vi "CMDExec.vi"() -> ()   [LabVIEW 2012]
uses:
  <vilib>/addons/database/Connection.llb/DB Tools Open Connec (String).vi
  <vilib>/Utility/file.llb/Read From Spreadsheet File (I64).vi
  <vilib>/Utility/file.llb/Read From Spreadsheet File (string).vi
  <vilib>/addons/database/NI_Database_API.lvlib
panel:
  in  "lot_end":string
  in  "lot_start":string
  out "output cluster":T1
  in  "input cluster":T1
  out "before substring 9":string
  out "concatenated string":string
  out "before substring":string
  out "standard output 3":string
  out "after substring":string
  out "text":string
  out "error out":errorcluster
  in  "error in (no error)":errorcluster
  out "standard error 2":string
  out "standard output 2":string
  out "standard error":string
  out "standard output":string
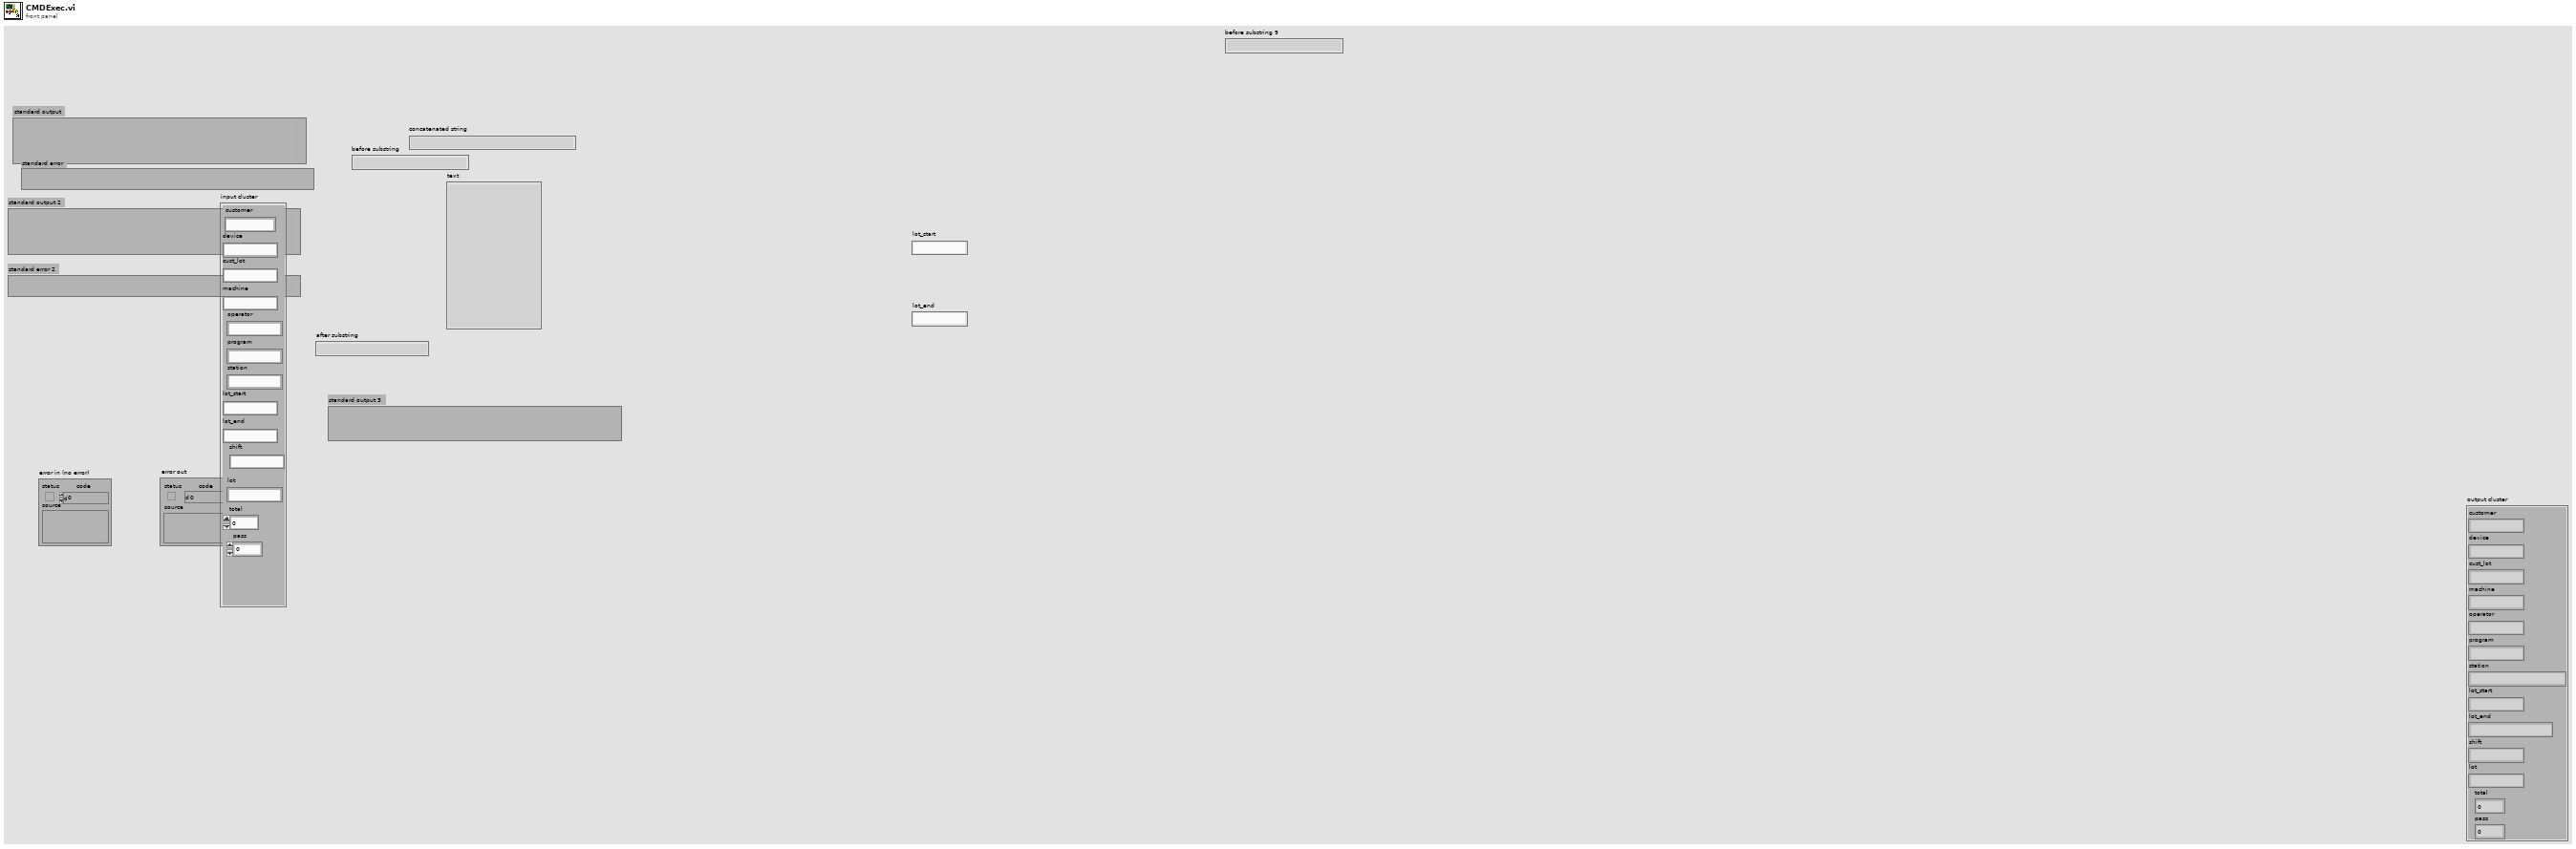
[diagram p1: front panel]
types:
  T1 = cluster{"customer":string, "device":string, "cust_lot":string, "machine":string, "operator":string, "program":string, "station":string, "lot_start":string, "lot_end":string, "shift":string, "lot":string, "total":dbl, "pass":dbl}
  T2 = enum16{"open", "replace", "create", "open or create", "replace or create", "replace or create with confirmation"}
  T3 = typedef "NI_Database_API.lvlib/Conn ObjectReference.ctl" = refnum<k1>
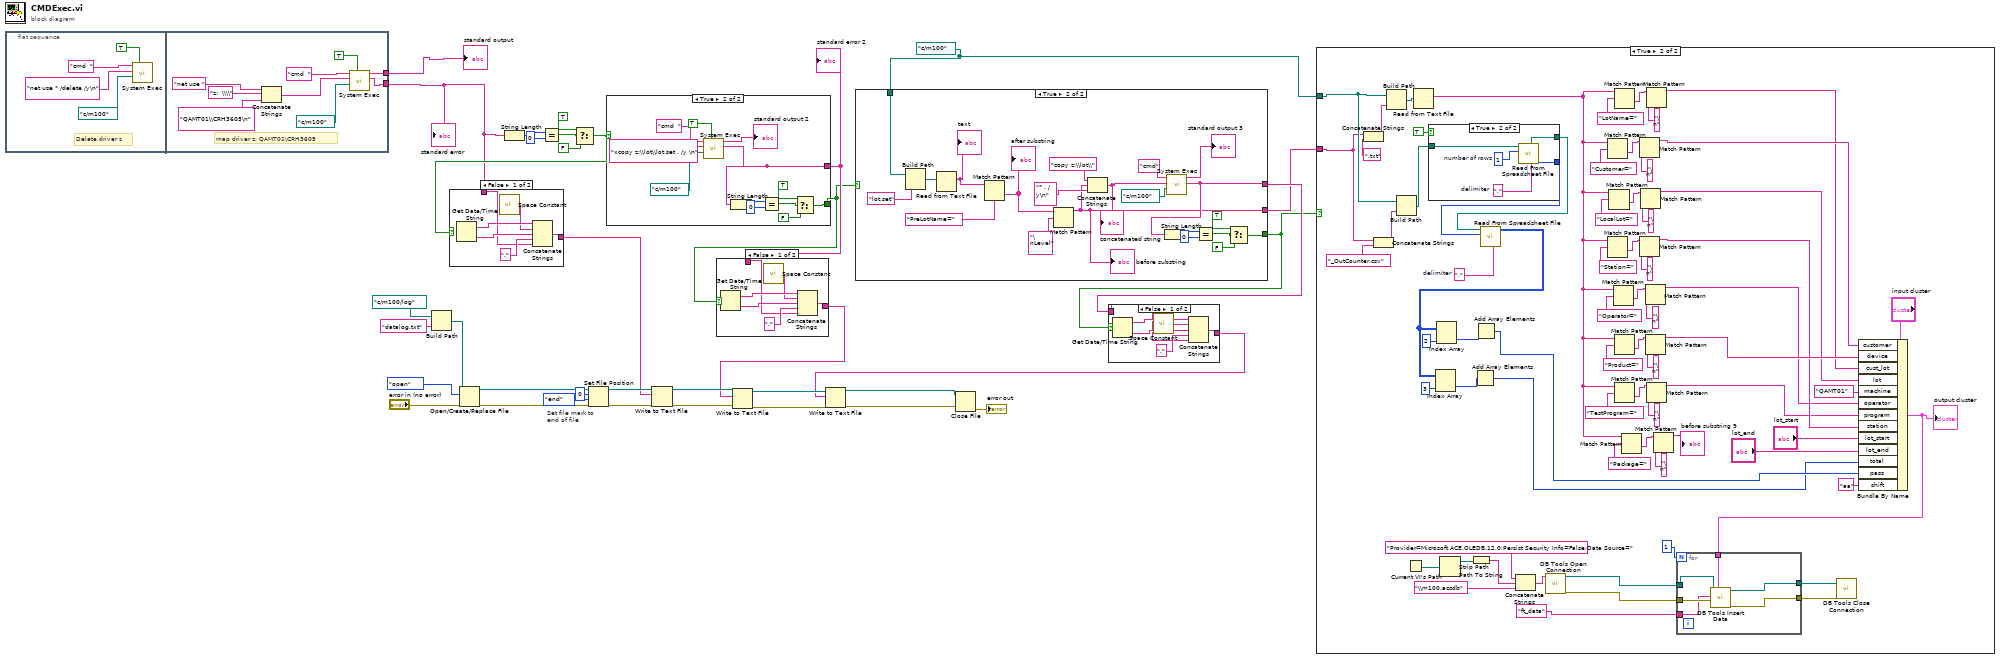
[diagram p0: block diagram]
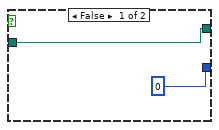
[diagram p3: hidden frame]
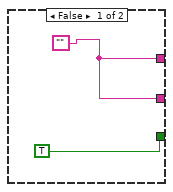
[diagram p5: hidden frame]
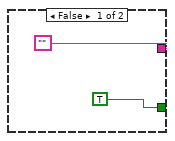
[diagram p8: hidden frame]
diagram:
  w2 = path "c:/m100" ("base path")
  # "Set file mark to\nend of file"
  n1 = flat-sequence {
    tunnel: [w41] -> w12
    tunnel: [w40] -> w11
    frame #0 {
      # "Delete driver z"
      n2 = call <vilib>:"System Exec.vi"("wait until completion? (T)"=TRUE, "working directory"=path "c:/m100", "standard input"="net use * /delete /y\n" ("string"), "command line"="cmd  ") -> ()  [unwired: 2 in, 6 out]
    }
    frame #1 {
      # "map driver z: QAMT01\\CRH3605"
      n3 = Concatenate Strings("net use " ("string"), "z:  \\\\" ("string"), "QAMT01\\CRH3605\n" ("string")) -> (w47:string)
      n4 = call <vilib>:"System Exec.vi"("wait until completion? (T)"=TRUE, "working directory"=path "c:/m100", "standard input"=w47, "command line"="cmd  ") -> ("standard error"=w40:string, "standard output"=w41:string)  [unwired: 2 in, 4 out]
    }
  }
  n5 = Build Path(base path=path "c:/m100/log" ("path"), name or relative path="datalog.txt") -> (appended path=w19:path)
  n6 = Open/Create/Replace File(file path (use dialog)=w19, error in="error in (no error)", operation (0:open)=T2."open") -> (refnum out=w24:refnum<file>, error out=w23:errorcluster)  [unwired: 3 in, 1 out]
  n7 = String Length(string=w11) -> (length=w35:i32)
  n8 = Equal?(x=w35, y=0) -> (x = y?=w33:bool)
  n9 = Select(t=TRUE, s=w33, f=FALSE) -> (s? t:f=w16:bool)
  n10 = case shown="False" w16 {
    tunnel: [w50 w55] -> w14
    tunnel: w11 -> [w49 w55]
    frame False {
      n11 = Get Date/Time String() -> (date string=w52:string, time string=w53:string)  [unwired: 3 in]
      n12 = call <vilib>:"Space Constant.vi"() -> ("String"=w51:string)
      n13 = Concatenate Strings(w52, w51, w53, "," ("string"), w49) -> (w50:string)
    }
    frame True {
    }
  }
  n14 = Set File Position(offset (in bytes) (0)=i64 0, refnum=w24, from (0:start)=enum16{"start", "end", "current"}."end", error in=w23) -> (refnum out=w26:refnum<file>, error out=w27:errorcluster)
  n15 = case shown="True" w16 {
    tunnel: [TRUE w59] -> w10
    tunnel: ["" w58] -> w15
    frame False {
    }
    frame True {
      n16 = call <vilib>:"System Exec.vi"("wait until completion? (T)"=TRUE, "working directory"=path "c:/m100", "standard input"="xcopy z:\\lot\\lot.set . /y \n", "command line"="cmd  ") -> ("standard error"=w58:string, "standard output"=→"standard output 2":string)  [unwired: 2 in, 4 out]
      n17 = String Length(string=w58) -> (length=w65:i32)
      n18 = Equal?(x=w65, y=0) -> (x = y?=w67:bool)
      n19 = Select(t=TRUE, s=w67, f=FALSE) -> (s? t:f=w59:bool)
    }
  }
  "standard error 2" <- w15
  n20 = Write to Text File(file (use dialog)=w26, text=w14, error in=w27) -> (refnum out=w18:refnum<file>, error out=w17:errorcluster)  [unwired: 1 in, 1 out]
  n21 = case shown="False" w10 {
    tunnel: [w71 w76] -> w13
    tunnel: w15 -> [w70 w76]
    frame False {
      n22 = Get Date/Time String() -> (date string=w73:string, time string=w74:string)  [unwired: 3 in]
      n23 = call <vilib>:"Space Constant.vi"() -> ("String"=w72:string)
      n24 = Concatenate Strings(w73, w72, w74, "," ("string"), w70) -> (w71:string)
    }
    frame True {
    }
  }
  n25 = Write to Text File(file (use dialog)=w18, text=w13, error in=w17) -> (refnum out=w6:refnum<file>, error out=w9:errorcluster)  [unwired: 1 in, 1 out]
  n26 = case shown="True" w10 {
    tunnel: [TRUE w83] -> w3
    tunnel: [w77 w82] -> w4
    tunnel: w2 -> [_ w80]
    tunnel: [w77 w79] -> w1
    frame False {
      w77 = ""
    }
    frame True {
      n27 = Build Path(base path=w80, name or relative path="lot.set") -> (appended path=w99:path)
      n28 = Read from Text File(file (use dialog)=w99) -> (text=w96:string)  [unwired: 3 in, 3 out]
      "text" <- w96
      n29 = Match Pattern(string=w96, regular expression="PreLotName=") -> (after substring=w90:string)  [unwired: 1 in, 3 out]
      "after substring" <- w90
      n30 = Match Pattern(string=w90, regular expression="\nLevel") -> (before substring=w79:string)  [unwired: 1 in, 3 out]
      "before substring" <- w79
      n31 = Concatenate Strings("copy z:\\lot\\" ("string"), w79, "* . /y\n" ("string")) -> (w89:string)
      "concatenated string" <- w89
      n32 = call <vilib>:"System Exec.vi"("working directory"=path "c:/m100", "standard input"=w89, "command line"="cmd") -> ("standard error"=w82:string, "standard output"=→"standard output 3":string)  [unwired: 3 in, 4 out]
      n33 = String Length(string=w82) -> (length=w84:i32)
      n34 = Equal?(x=w84, y=0) -> (x = y?=w86:bool)
      n35 = Select(t=TRUE, s=w86, f=FALSE) -> (s? t:f=w83:bool)
    }
  }
  n36 = case shown="False" w3 {
    tunnel: [w101 w106] -> w5
    tunnel: w4 -> [w100 w106]
    frame False {
      n37 = Get Date/Time String() -> (date string=w103:string, time string=w104:string)  [unwired: 3 in]
      n38 = call <vilib>:"Space Constant.vi"() -> ("String"=w102:string)
      n39 = Concatenate Strings(w103, w102, w104, "," ("string"), w100) -> (w101:string)
    }
    frame True {
    }
  }
  n40 = Write to Text File(file (use dialog)=w6, text=w5, error in=w9) -> (refnum out=w8:refnum<file>, error out=w7:errorcluster)  [unwired: 1 in, 1 out]
  n41 = Close File(refnum=w8, error in=w7) -> (error out=→"error out":errorcluster)  [unwired: 1 out]
  n42 = case shown="True" w3 {
    tunnel: w2 -> [_ w108]
    tunnel: w1 -> [_ w107]
    frame False {
    }
    frame True {
      w145 = ","  # delimiter
      n43 = Concatenate Strings(w107, ".txt" ("string")) -> (w176:string)
      n44 = Concatenate Strings(w107, "_OutCounter.csv" ("string")) -> (w147:string)
      n45 = Build Path(base path=w108, name or relative path=w176) -> (appended path=w173:path)
      n46 = Build Path(base path=w108, name or relative path=w147) -> (appended path=w139:path)
      n47 = Current VI's Path() -> (path=w135:path)
      n48 = Read from Text File(file (use dialog)=w173) -> (text=w148:string)  [unwired: 3 in, 3 out]
      n49 = case shown="True" TRUE {
        tunnel: [0 ("mark after read (chars.)") w185] -> w137
        tunnel: [w184 w187] -> w138
        tunnel: w139 -> [w184 w186]
        frame False {
        }
        frame True {
          w188 = 1  # number of rows
          w189 = ","  # delimiter
          n50 = call-poly <vilib>:"Read From Spreadsheet File.vi"("delimiter (\\t)"=w189, "number of rows (all:-1)"=w188, "file path (dialog if empty)"=w186) -> ("mark after read (chars.)"=w185:i32, "new file path (Not A Path if cancelled)"=w187:path)  [unwired: 4 in, 3 out]
        }
      }
      n51 = Strip Path(path=w135) -> (stripped path=w134:path)  [unwired: 1 out]
      n52 = Path To String(path=w134) -> (string=w133:string)
      n53 = call-poly <vilib>:"Read From Spreadsheet File.vi"("delimiter (\\t)"=w145, "number of rows (all:-1)"=w137, "file path (dialog if empty)"=w138) -> ("all rows"=w140:i64[][])  [unwired: 4 in, 4 out]
      n54 = Index Array(array=w140, index (col)=3 ("disabled index (col)")) -> (element=w141:i64[])  [unwired: 1 in]
      n55 = Index Array(array=w140, index (col)=2 ("disabled index (col)")) -> (element=w143:i64[])  [unwired: 1 in]
      n56 = Add Array Elements(numeric array=w141) -> (sum=w119:i64)
      n57 = Add Array Elements(numeric array=w143) -> (sum=w120:i64)
      n58 = Concatenate Strings("Provider=Microsoft.ACE.OLEDB.12.0;Persist Security Info=False;Data Source=", w133, "\\m100.accdb") -> (w131:string)
      n59 = call-poly <vilib>:"DB Tools Open Connection.vi"("connection information"=w131) -> ("error out"=w116:errorcluster, "connection reference"=w117:T3)  [unwired: 7 in]
      n60 = Match Pattern(string=w148, regular expression="Customer=") -> (after substring=w169:string)  [unwired: 1 in, 3 out]
      n61 = Match Pattern(string=w148, regular expression="Station=") -> (after substring=w163:string)  [unwired: 1 in, 3 out]
      n62 = Match Pattern(string=w148, regular expression="LocalLot=") -> (after substring=w166:string)  [unwired: 1 in, 3 out]
      n63 = Match Pattern(string=w148, regular expression="Operator=") -> (after substring=w160:string)  [unwired: 1 in, 3 out]
      n64 = Match Pattern(string=w148, regular expression="Product=") -> (after substring=w157:string)  [unwired: 1 in, 3 out]
      n65 = Match Pattern(string=w148, regular expression="LotName=") -> (after substring=w172:string)  [unwired: 1 in, 3 out]
      n66 = Match Pattern(string=w148, regular expression="TestProgram=") -> (after substring=w154:string)  [unwired: 1 in, 3 out]
      n67 = Match Pattern(string=w148, regular expression="Package=") -> (after substring=w151:string)  [unwired: 1 in, 3 out]
      n68 = Match Pattern(string=w169, regular expression="\n") -> (before substring=w127:string)  [unwired: 1 in, 3 out]
      n69 = Match Pattern(string=w163, regular expression="\n") -> (before substring=w123:string)  [unwired: 1 in, 3 out]
      n70 = Match Pattern(string=w166, regular expression="\n") -> (before substring=w124:string)  [unwired: 1 in, 3 out]
      n71 = Match Pattern(string=w160, regular expression="\n") -> (before substring=w122:string)  [unwired: 1 in, 3 out]
      n72 = Match Pattern(string=w157, regular expression="\n") -> (before substring=w126:string)  [unwired: 1 in, 3 out]
      n73 = Match Pattern(string=w172, regular expression="\n") -> (before substring=w125:string)  [unwired: 1 in, 3 out]
      n74 = Match Pattern(string=w154, regular expression="\n") -> (before substring=w121:string)  [unwired: 1 in, 3 out]
      n75 = Match Pattern(string=w151, regular expression="\n") -> (before substring=→"before substring 9":string)  [unwired: 1 in, 3 out]
      n76 = Bundle By Name(cluster="input cluster", "customer"=w127, "device"=w126, "cust_lot"=w125, "lot"=w124, "machine"="QAMT01", "operator"=w122, "program"=w121, "station"=w123, "lot_start"="lot_start", "lot_end"="lot_end", "total"=w119, "pass"=w120, "shift"="aa") -> (w128:T1)
      "output cluster" <- w128
      n77 = for {
        N: 1 -> [_]
        tunnel: w128 -> [w182]
        tunnel: w117 -> [w181]
        tunnel: w116 -> [w180]
        tunnel: [w179] -> w111
        tunnel: "ft_data" ("table") -> [w178]
        tunnel: [w177] -> w110
        n78 = call <vilib>:"DB Tools Insert Data.vi"("data"=w182, "error in (no error)"=w180, "table"=w178, "connection reference"=w181) -> ("error out"=w179:errorcluster, "connection reference out"=w177:T3)  [unwired: 6 in]
      }
      n79 = call <vilib>:"DB Tools Close Connection.vi"("error in (no error)"=w111, "connection reference"=w110) -> ()  [unwired: 5 in, 1 out]
    }
  }
  "standard output" <- w12
  "standard error" <- w11
